vi "DriveUntilY.vi"(8 "error in":errorcluster, 9 "y":dbl, 10 "x":dbl, 11 "y-axis distance":dbl) -> (0 "error out":errorcluster)   [LabVIEW 2017]
uses:
  <vilib>/Rock Robotics/WPI/Ultrasonic/WPI_SonarSRF04DigitalRefNum Registry Get.vi
  <vilib>/Rock Robotics/WPI/Ultrasonic/WPI_SonarSRF04DigitalGetRange.vi
  Robot Global Data.vi
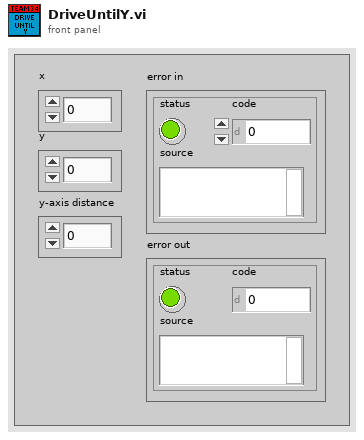
[diagram p1: front panel]
types:
  T1 = typedef "WPI_UltrasonicDeviceRef.ctl" = cluster{"DevStatus":errorcluster, "Ping Channel":T2, "Echo Channel":T2, "CntIndex":T3}
  T2 = typedef "FPGA_DIOChannel.ctl" = enum8{"DIO 0", "DIO 1", "DIO 2", "DIO 3", "DIO 4", "DIO 5", "DIO 6", "DIO 7", "DIO 8", "DIO 9", "DIO MXP 0", "DIO MXP 1", "DIO MXP 2", "DIO MXP 3", "DIO MXP 4", "DIO MXP 5", "DIO MXP 6", "DIO MXP 7", "DIO MXP 8", "DIO MXP 9", "DIO MXP 10", "DIO MXP 11", "DIO MXP 12", "DIO MXP 13", "DIO MXP 14", "DIO MXP 15", "SPI Port CS1", "SPI Port CS2", "SPI Port CS3", "SPI Port MISO", "SPI Port MOSI", "Invalid"}
  T3 = typedef "FPGA_CounterCtrSystemIndex.ctl" = enum8{"Ctr 0", "Ctr 1", "Ctr 2", "Ctr 3", "Ctr 4", "Ctr 5", "Ctr 6", "Ctr 7", "Invalid"}
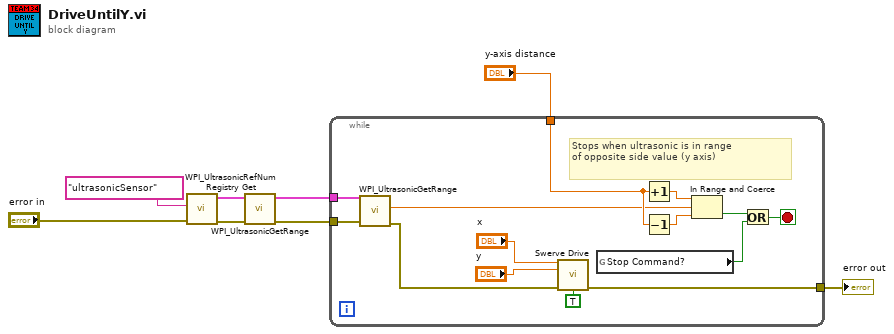
[diagram p0: block diagram]
diagram:
  n1 = call-poly <vilib>:"WPI_UltrasonicRefNum Registry Get.vi"("error in (no error)"="error in", "refnum name"="ultrasonicSensor") -> ("error out"=w2:errorcluster, "SonarSRF04DevRef"=w1:T1)  [unwired: 8 in]
  n2 = call-poly <vilib>:"WPI_UltrasonicGetRange.vi"("error in (no error)"=w2, "SonarSRF04DevRef"=w1) -> ("error out"=w4:errorcluster, "SonarSRF04DevRef"=w5:T1)  [unwired: 7 in, 1 out]
  n3 = while {
    tunnel: w4 -> [w21]
    tunnel: w5 -> [w22]
    tunnel: [w13] -> w6
    tunnel: "y-axis distance" -> [w12]
    stop <- w16 stop-if-true
    # "Stops when ultrasonic is in range\nof opposite side value (y axis)"
    n4 = call-poly <vilib>:"WPI_UltrasonicGetRange.vi"("error in (no error)"=w21, "SonarSRF04DevRef"=w22) -> ("error out"=w15:errorcluster, "Distance"=w11:dbl)  [unwired: 7 in, 1 out]
    n5 = call "Swerve Drive.vi"("X"="x", "Y"="y", "Error In"=w15, "Autonomous?"=TRUE) -> ("Error Out"=w13:errorcluster)  [unwired: 7 in, 4 out]
    n6 = global read "Robot Global Data.vi" "Stop Command?"() -> (w17:bool)
    n7 = Increment(x=w12) -> (x+1=w20:dbl)
    n8 = Decrement(x=w12) -> (x-1=w19:dbl)
    n9 = In Range and Coerce(upper limit=w20, x=w11, lower limit=w19) -> (In Range?=w18:bool)  [unwired: 1 out]
    n10 = Or(x=w18, y=w17) -> (x .or. y?=w16:bool)
  }
  "error out" <- w6
